vi "test_AM.vi"() -> ()   [LabVIEW 2013]
panel:
  out "size(s)":i32
  in  "Upper chart":dbl[][](graph)
  out "Numeric":i32
  out "Waveform Graph":dbl[][](graph)
  in  "Data in":fxp<+/-,16,14>[](array[numeric])=[0.0, 0.0, 0.0, 0.0]
  in  "Output delay delta":dbl(slide) scale=0.0..6.0
  in  "Output delay":dbl(slide) scale=0.0..6.0
  in  "Mixer freq [MHz]":dbl
  in  "b_am":fxp<+/-,16,2>
  in  "a_am":fxp<+/-,16,2>
  in  "Am freq [kHz]":dbl=10.0
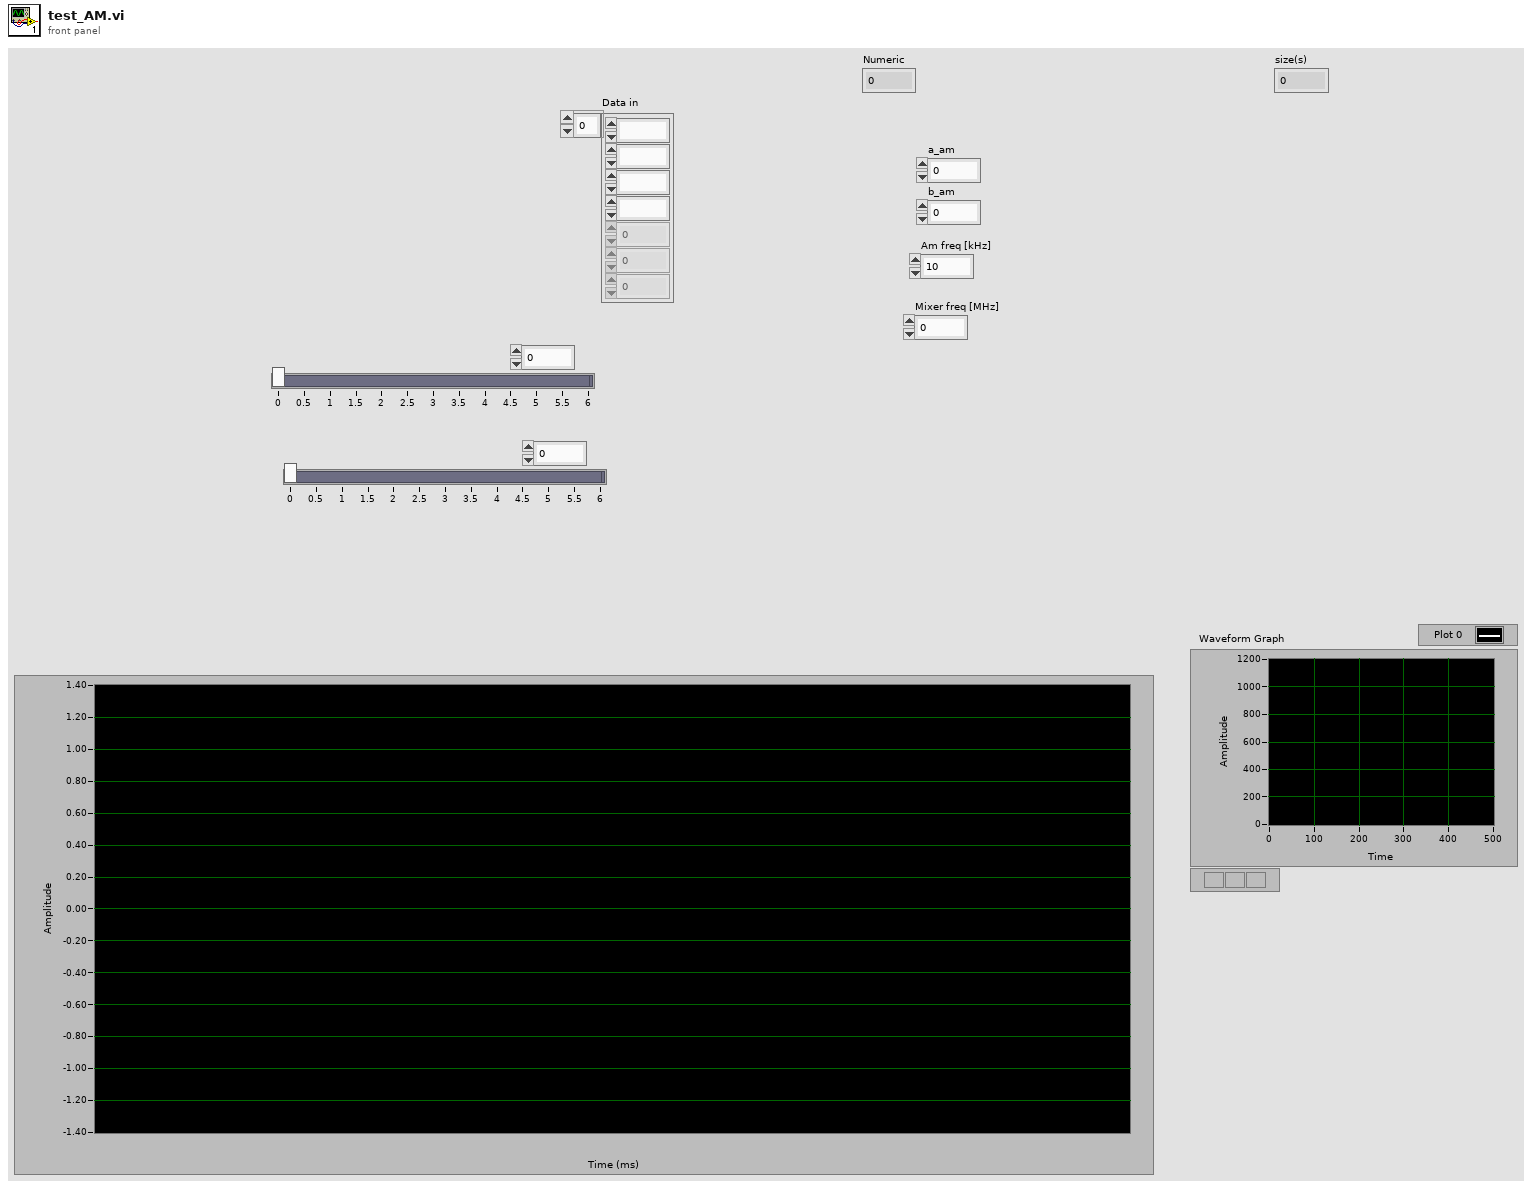
[diagram p1: front panel]
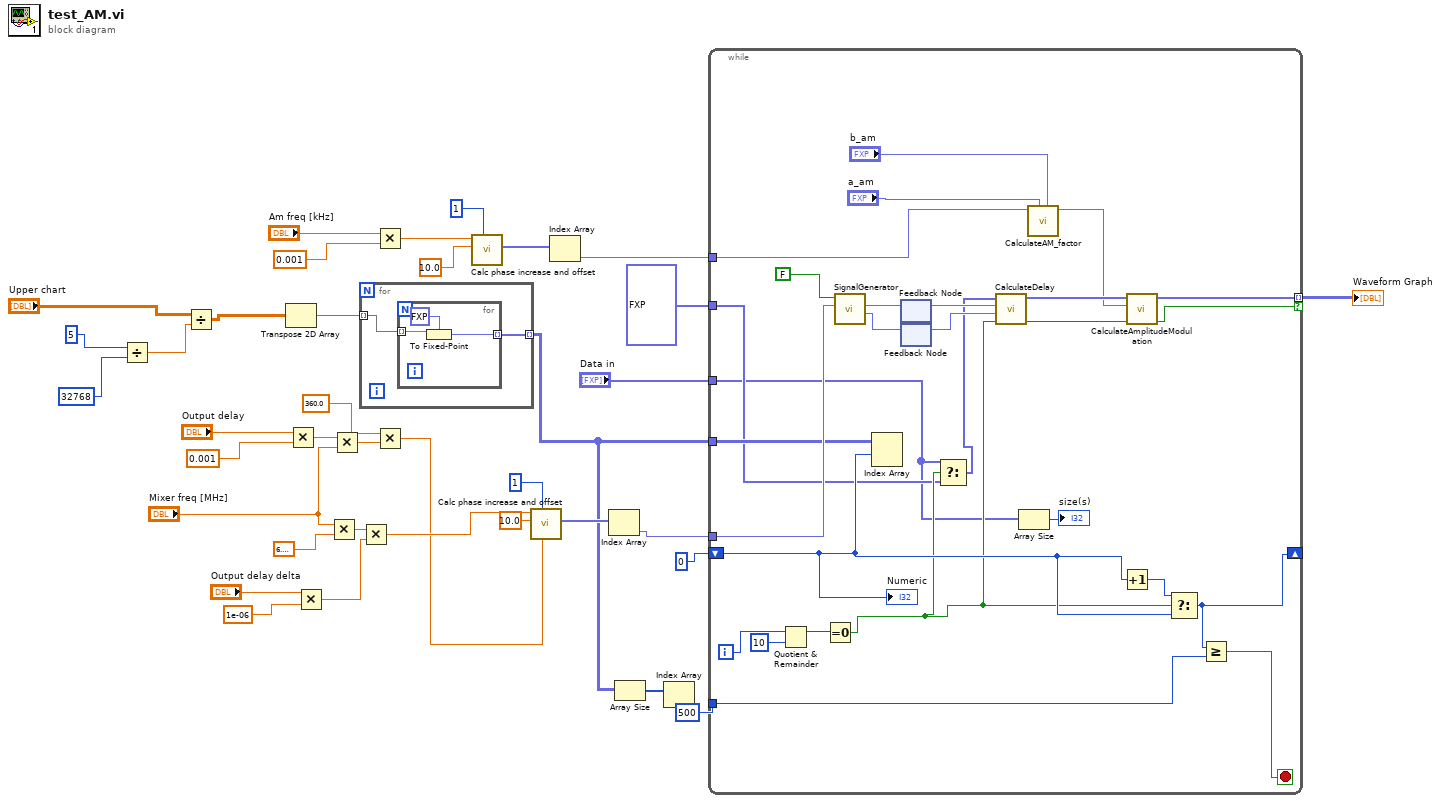
[diagram p0: block diagram]
diagram:
  n1 = Divide(x=5, y=32768) -> (x/y=w7:dbl)
  n2 = Divide(x="Upper chart", y=w7) -> (x/y=w6:dbl[][])
  n3 = Transpose 2D Array(2D array=w6) -> (transposed array=w11:dbl[][])
  n4 = Multiply(x="Output delay", y=0.001) -> (x*y=w20:dbl)
  n5 = Multiply(x="Output delay delta", y=1e-06) -> (x*y=w22:dbl)
  n6 = Multiply(x="Mixer freq [MHz]", y=6.283185307179586) -> (x*y=w27:dbl)
  n7 = Multiply(x=w20, y="Mixer freq [MHz]") -> (x*y=w19:dbl)
  n8 = for {
    tunnel: w11 -> [w39] mode=indexing
    tunnel: [w38] -> w3 mode=indexing
    n9 = for {
      tunnel: w39 -> [w42] mode=indexing
      tunnel: [w40] -> w38 mode=indexing
      n10 = To Fixed-Point(fixed-point type=fxp<+/-,16,14> 0.0 ("Q in"), number=w42) -> (fixed-point=w40:fxp<+/-,16,14>)
    }
  }
  n11 = Multiply(x=w27, y=w22) -> (x*y=w26:dbl)
  n12 = Multiply(x="Am freq [kHz]", y=0.001) -> (x*y=w32:dbl)
  n13 = Multiply(x=360.0, y=w19) -> (x*y=w17:dbl)
  n14 = call "Calc phase increase and offset.vi"("# of DDS"=1, "fclk (MHz)"=10.0, "f_generated (MHz)"=w32) -> ("Phase out"=w33:fxp<+,64,64>[])  [unwired: 6 in, 2 out]
  n15 = call "Calc phase increase and offset.vi"("Phase offset (deg)"=w17, "# of DDS"=1, "fclk (MHz)"=10.0, "f_generated (MHz)"=w26) -> ("Phase out"=w16:fxp<+,64,64>[])  [unwired: 5 in, 2 out]
  n16 = Index Array(array=w33) -> (element=w31:fxp<+,64,64>)  [unwired: 1 in]
  n17 = Index Array(array=w16) -> (element=w15:fxp<+,64,64>)  [unwired: 1 in]
  n18 = Array Size(array=w3) -> (size(s)=w4:i32[])
  n19 = Index Array(array=w4) -> ()  [unwired: 1 in, 1 out]
  n20 = while {
    tunnel: w31 -> [w44]
    tunnel: w15 -> [w67]
    tunnel: "Data in" -> [w47]
    tunnel: [w63] -> w13 mode=indexing if=w62
    tunnel: w3 -> [w58]
    shift-right: [w56] -> _
    shift-left: 0 ("y") -> [w53]
    tunnel: 500 -> [w55]
    tunnel: fxp<+/-,16,14>[] [0.0, 0.0, 0.0, 0.0] ("f") -> [w49]
    i -> [w66]
    stop <- w54 stop-if-true
    n21 = Quotient & Remainder(x=w66, y=10) -> (x-y*floor(x/y)=w64:i32)  [unwired: 1 out]
    n22 = Equal To 0?(x=w64) -> (x = 0?=w50:bool)
    n23 = call "SignalGenerator.vi"("phase"=w67, "Reset"=FALSE) -> ("Cos"=w68:fxp<+/-,16,0>, "Sin"=w69:fxp<+/-,16,0>)  [unwired: 7 in, 1 out]
    n24 = Index Array(array=w58, index (row)=w53) -> ()  [unwired: 1 in, 1 out]
    n25 = feedback #1() -> (w59:fxp<+/-,16,0>)  [unwired: 1 in]
    n26 = feedback-in #1(w69) -> ()
    n27 = feedback #2() -> (w60:fxp<+/-,16,0>)  [unwired: 1 in]
    n28 = feedback-in #2(w68) -> ()
    n29 = Select(t=w47, s=w50, f=w49) -> (s? t:f=w48:fxp<+/-,16,14>[])
    n30 = call "CalculateDelay.vi"("input valid"=w50, "cos_fi"=w60, "sin fi"=w59, "Data in"=w48) -> ("output valid"=w51:bool, "Data out"=w52:fxp<+/-,16,14>[])  [unwired: 6 in]
    n31 = Array Size(array=w47) -> (size(s)=→"size(s)":i32)
    n32 = call "CalculateAM_factor.vi"("b_am"="b_am", "a_am"="a_am", "AM phase"=w44) -> ("AM_factor"=w43:fxp<+/-,16,2>)  [unwired: 7 in, 1 out]
    n33 = Increment(x=w53) -> (x+1=w57:i32)
    n34 = call "CalculateAmplitudeModulation.vi"("input valid"=w51, "AM_factor"=w43, "Data in"=w52) -> ("output valid"=w62:bool, "Data out"=w63:fxp<+/-,16,14>[])  [unwired: 7 in]
    n35 = Select(t=w57, s=w50, f=w53) -> (s? t:f=w56:i32)
    n36 = Greater Or Equal?(x=w56, y=w55) -> (x >= y?=w54:bool)
    "Numeric" <- w53
  }
  "Waveform Graph" <- w13
